vi "CUENTA_FINAL.vi"(8 "error in (no error)":errorcluster, 10 "event data":bool[](array[boolean]), 11 "CONTEO_DIG in":refnum<class "CONTEO_DIG.lvclass">) -> (0 "error out":errorcluster, 3 "CONTEO_DIG out":refnum<class "CONTEO_DIG.lvclass">)   [LabVIEW 2019, in "CONTEO_DIG.lvlib" / "CONTEO_DIG.lvclass"]
uses:
  CONTEO_DIG.lvclass
  CONTEO_DIG.lvclass/CONTEO_DIG.ctl
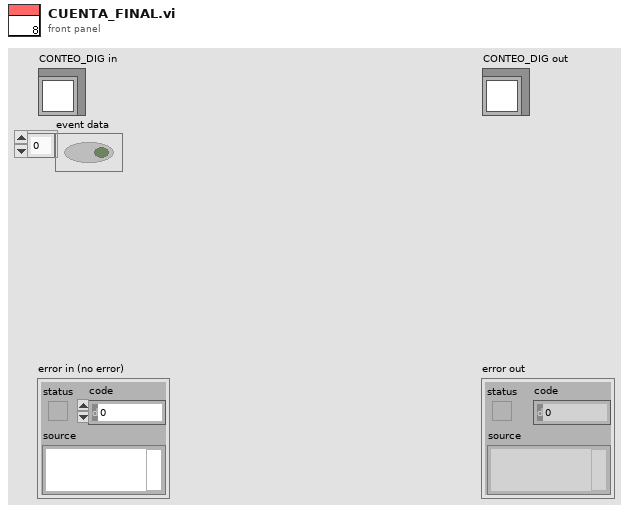
[diagram p1: front panel]
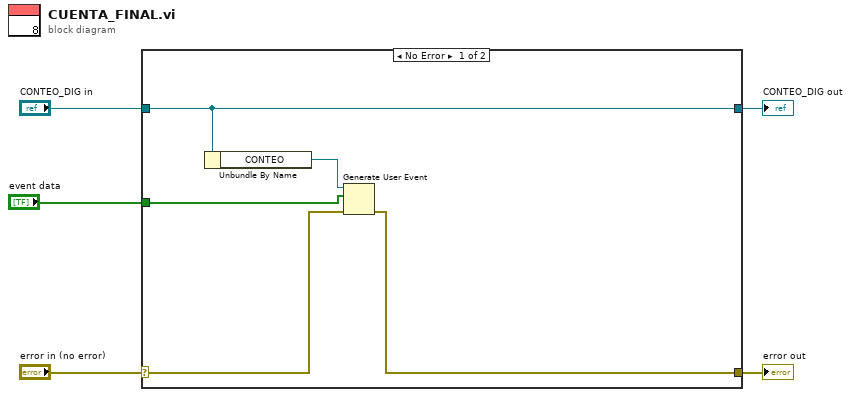
[diagram p0: block diagram]
diagram:
  n1 = case shown="No Error" "error in (no error)" {
    selector: "error in (no error)" -> [w7 w12]
    tunnel: [w6 w12] -> w4
    tunnel: [w10 w11] -> w2
    tunnel: "CONTEO_DIG in" -> [w10 w11]
    tunnel: "event data" -> [w8 _]
    frame No Error {
      n2 = Unbundle By Name(w10) -> ("CONTEO"=w9:refnum<user-event>)
      n3 = Generate User Event(user event=w9, event data cluster=w8, error in=w7) -> (error out=w6:errorcluster)  [unwired: 1 in, 1 out]
    }
    frame Error {
    }
  }
  "error out" <- w4
  "CONTEO_DIG out" <- w2
